vi "Example_OE2031&OE2041 Control.vi"() -> ()   [LabVIEW 2011]
uses:
  <vilib>/Utility/error.llb/DialogType.ctl
panel:
  in  "Sample count":u32
  out "Zero Data?":bool
  in  "buffer":u8
  out "Queue out":errorcluster caption="error out"
  out "Queue output":refnum<queue>
  in  "IP Address":string
  in  "Timeout":u32=100
  in  "Port":u32=10001
  out "Gain Overlaod":bool
  in  "Remote Mode":u16(ring) items=["USB"=0, "RS232"=1, "Ethernet"=3]
  out "Freq":dbl
  out "xita":dbl
  out "R":dbl
  out "Input Overlaod":bool
  out "PLL Lock":bool
  out "Error":string
  out "Serial Versions":string
  in  "Table":T1(tab) caption="选项卡控件"
  in  "OE2041_Configure Input Filter":T2 {"Input Impedance" items=["50Ω", "10MΩ"]; "Input Coupling" items=["AC", "DC"]; "Input Shield Grounding" items=["Float", "Ground"]; "Input Source" items=["A", "B"]}
  in  "OE2041_Configure Ref Phase":T3={"Reference Source"=0, "Sweep Mode"=0, "Start Frequency"=1000.0, "Stop Frequency"=5000.0, "Linear Step Frequency"=1000.0, "Log Step Percent"=10.0, "Step Time(ms)"=1000, "Sweep Run Mode"=0, "Internal Frequency"=1000.0, "Phase  (degree)"=0.0, "External Ref Trigger"=0, "Instrument Mode "=8} {"Instrument Mode" items=["OE2031-10M"=6, "OE2041-30M"=7, "OE2041-60M"=8]; "External Ref Trigger" items=["TTL Rising Edge", "Sine Zero Crossing"]; "Phase  (degree)" min=-180.0 max=180.0 format="%#.2g"; "Internal Frequency" min=1e-05 max=60000000.0 format="%#.3f"; "Sweep Run Mode" items=["Stop", "Singal", "Loop"]; "Log Step Percent" min=-100.0 max=100.0 format="%#.2f"; "Linear Step Frequency" min=1e-05 max=60000000.0 format="%#.3f"; "Stop Frequency" min=1e-05 max=60000000.0 format="%#.3f"; "Start Frequency" min=1e-05 max=60000000.0 format="%#.3f"; "Sweep Mode" items=["Linear", "Log"]; "Reference Source" items=["External", "Internal", "Internal Sweep", "Self"]}
  in  "OE2041_Configure Sens and Filter":T4={"Input Range"=0, "Sensitivity "=24, "Time Constant "=20, "Low Pass Filter Slope "=3, "Enable Sync Filter "=0} {"Enable Sync Filter" items=["OFF", "ON"]; "Low Pass Filter Slope" items=["6 dB/oct", "12 dB/oct", "18 db/oct", "24 dB/oct", "30 dB/oct", "36 dB/oct", "42 dB/oct", "48 dB/oct"]; "Time Constant" items=["30 ns", "60 ns", "125 ns", "250 ns", "500 ns", "1 us", "2 us", "4 us", "8 us", "16 us", "32 us", "64 us", "125 us", "250 us", "500 us", "1 ms", "2 ms", "4 ms", "8 ms", "16 ms", "32 ms", "65 ms", "125 ms", "250 ms", "500 ms", "1 s", "2 s", "4 s", "8 s", "17 s", "35 s", "70 s", "140 s", "275 s", "550 s", "1100 s", "2200 s", "4400 s"]; "Sensitivity" items=["1 nV/fA", "2 nV/fA", "5 nV/fA", "10 nV/fA", "20 nV/fA", "50 nV/fA", "100 nV/fA", "200 nV/fA", "500 nV/fA", "1 uV/pA", "2 uV/pA", "5 uV/pA", "10 uV/pA", "20 uV/pA", "50 uV/pA", "100 uV/pA", "200 uV/pA", "500 uV/pA", "1 mV/nA", "2 mV/nA", "5 mV/nA", "10 mV/nA", "20 mV/nA", "50 mV/nA", "100 mV/nA", "200 mV/nA", "500 mV/nA", "1 V/uA"]; "Input Range" items=["1V", "200mV", "50mV", "10mV", "2mV", "400uV"]}
  in  "OE2041_Configure Channel Out":T5={"parameter"=0, "Speed"=0, "Offset(%)"=0.0, "Expand"=1.0, "AUX OUT"=1.0, "Channel"=0} {"Channel" items=["CH1", "CH2", "CH3", "CH4"]; "AUX OUT" min=-10.0 max=10.0 format="%#.3g"; "Expand" min=1.0 max=256.0 format="%#_3g"; "Offset(%)" min=-100.0 max=100.0 format="%#_5g"; "Speed" items=["Slow", "Fast"]; "parameter" items=["AUXOUT", "X", "Y", "R", "Theta", "Xh1", "Yh1", "Rh1", "Theta h1", "Xh2", "Yh2", "Rh2", "Theta h2", "Xh3", "Yh3", "Rh3", "Theta h3", "X_Noise", "Y_Noise", "Frequency", "AUX-IN1", "AUX-IN2", "AUX-IN3", "AUX-IN4"]}
  in  "OE2041_Configure Sine Out":T6={"Start Value(V)"=0.1, "Sine Output Amplitude (V)"=1.0, "Stop Valve(V)"=1.0, "Sine Step Valve(V)"=0.1, "Step Time(ms) "=1000, "Sine Step Percent(%)"=10.0, "SineOut Mode"=0, "Sine Run Mode"=0, "ADD Mode"=0} {"ADD Mode" items=["OFF", "ON"]; "Sine Run Mode" items=["Stop", "Single", "Loop"]; "SineOut Mode" items=["OFF", "Fixed", "Linear", "Log"]; "Sine Step Percent(%)" min=0.0 max=100.0 format="%#.2g"; "Step Time(ms)" min=1 max=100000; "Sine Step Valve(V)" min=1e-06 max=1.0 format="%#.3g"; "Stop Valve(V)" min=1e-06 max=1.0 format="%#.3g"; "Sine Output Amplitude (V)" min=0.001 max=1.0 format="%#.3g"; "Start Value(V)" min=1e-06 max=1.0 format="%#.3g"}
  in  "OE2041_Configure Demodulator":T7={"A"=1, "F1"=1.0, "B"=1, "F2"=1.0, "Demodulator"=1, "Mode"=0, "Arbitrary Frequency"=1000.0, "Harmonic"=1, "Instrument Mode "=8} {"Instrument Mode" items=["OE2031-10M"=6, "OE2041-30M"=7, "OE2041-60M"=8]; "Harmonic" min=1 max=32767; "Arbitrary Frequency" min=1e-05 max=60000000.0 format="%#.3f"; "Mode" items=["Harm", "Arb_Freq", "Equation"]; "Demodulator" items=["1", "2", "3"]; "F2" min=1e-05 max=60000000.0 format="%#.3g"; "B" min=-32767; "F1" min=1e-05 max=60000000.0 format="%#.3g"; "A" min=-32767}
  in  "OE2041_Auto Setting":T8
  in  "Save Button":bool
  in  "file path":path
  in  "Sample Rate":dbl=0.1 min=0.001 max=100.0
  out "Status":string
  in  "Connect":bool
  in  "VISA resource name":refnum<visa-resource-name>
  in  "Baud Rate (921600)":u32=921600
  # "Tel          :   +86-020-84133345\nWebsite  :   www.ssi-instrument.com\nE-mail     :   support@si-instrument.com"
  # "E="
  # "×"
  # "+"
  # "×"
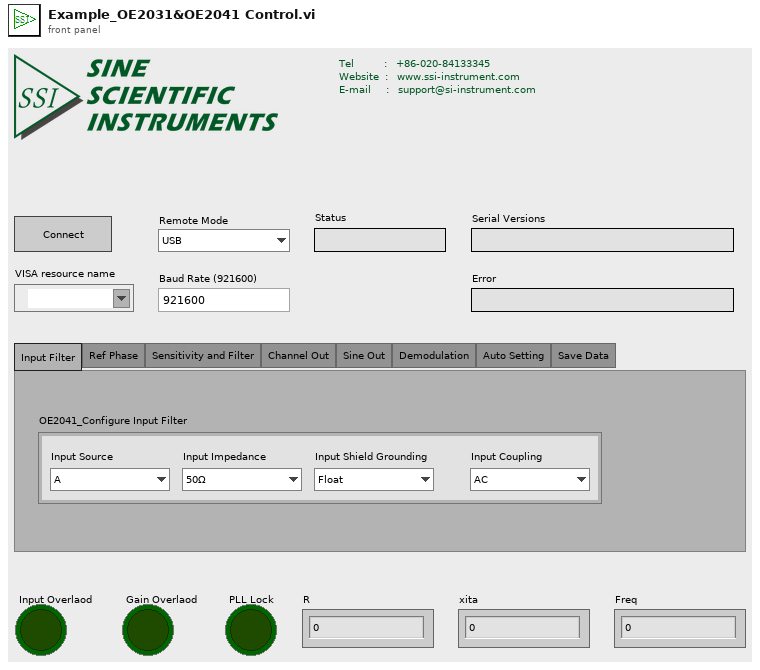
[diagram p1: front panel]
types:
  T1 = enum32{"Input Filter", "Ref Phase", "Sensitivity and Filter", "Channel Out", "Sine Out", "Demodulation", "Auto Setting", "Save Data"}
  T2 = cluster{"Input Source":u16, "Input Shield Grounding ":u16, "Input Coupling ":u16, "Input Impedance ":u16}
  T3 = cluster{"Reference Source":u16, "Sweep Mode":u16, "Start Frequency":dbl, "Stop Frequency":dbl, "Linear Step Frequency":dbl, "Log Step Percent":dbl, "Step Time(ms)":i32, "Sweep Run Mode":u16, "Internal Frequency":dbl, "Phase  (degree)":dbl, "External Ref Trigger":u16, "Instrument Mode ":u16}
  T4 = cluster{"Input Range":u16, "Sensitivity ":u16, "Time Constant ":u8, "Low Pass Filter Slope ":u8, "Enable Sync Filter ":u16}
  T5 = cluster{"parameter":u16, "Speed":u16, "Offset(%)":dbl, "Expand":dbl, "AUX OUT":dbl, "Channel":u16}
  T6 = cluster{"Start Value(V)":dbl, "Sine Output Amplitude (V)":dbl, "Stop Valve(V)":dbl, "Sine Step Valve(V)":dbl, "Step Time(ms) ":u32, "Sine Step Percent(%)":dbl, "SineOut Mode":u8, "Sine Run Mode":u8, "ADD Mode":u8}
  T7 = cluster{"A":i16, "F1":dbl, "B":i16, "F2":dbl, "Demodulator":u16, "Mode":u16, "Arbitrary Frequency":dbl, "Harmonic":u16, "Instrument Mode ":u16}
  T8 = cluster{"Auto Gain":bool, "Auto Phase":bool, "Auto Scale":bool}
  T9 = enum16{"OE1022", "OE1022D", "OE1201", "OE2031&OE2041", "OE1311&OE1351"}
  T10 = cluster{"Port":u32, "Timeout":u32, "IP Address":string}
  T11 = cluster{"PLL Lock(1: External Lock)":bool, "Input Overlaod":bool, "Gain Overlaod":bool}
  T12 = cluster{"X":dbl, "Y":dbl, "R":dbl, "θ":dbl, "Frequency":dbl, "XD1":dbl, "YD1":dbl, "RD1":dbl, "θD1":dbl, "XD2":dbl, "YD2":dbl, "RD2":dbl, "θD2":dbl, "XD3":dbl, "YD3":dbl, "RD3":dbl, "θD3":dbl, "X-Noise":dbl, "Y-Noise":dbl, "AUX-IN1":dbl, "AUX-IN2":dbl, "AUX-IN3":dbl, "AUX-IN4":dbl}
  T13 = typedef "DialogType.ctl" = u16
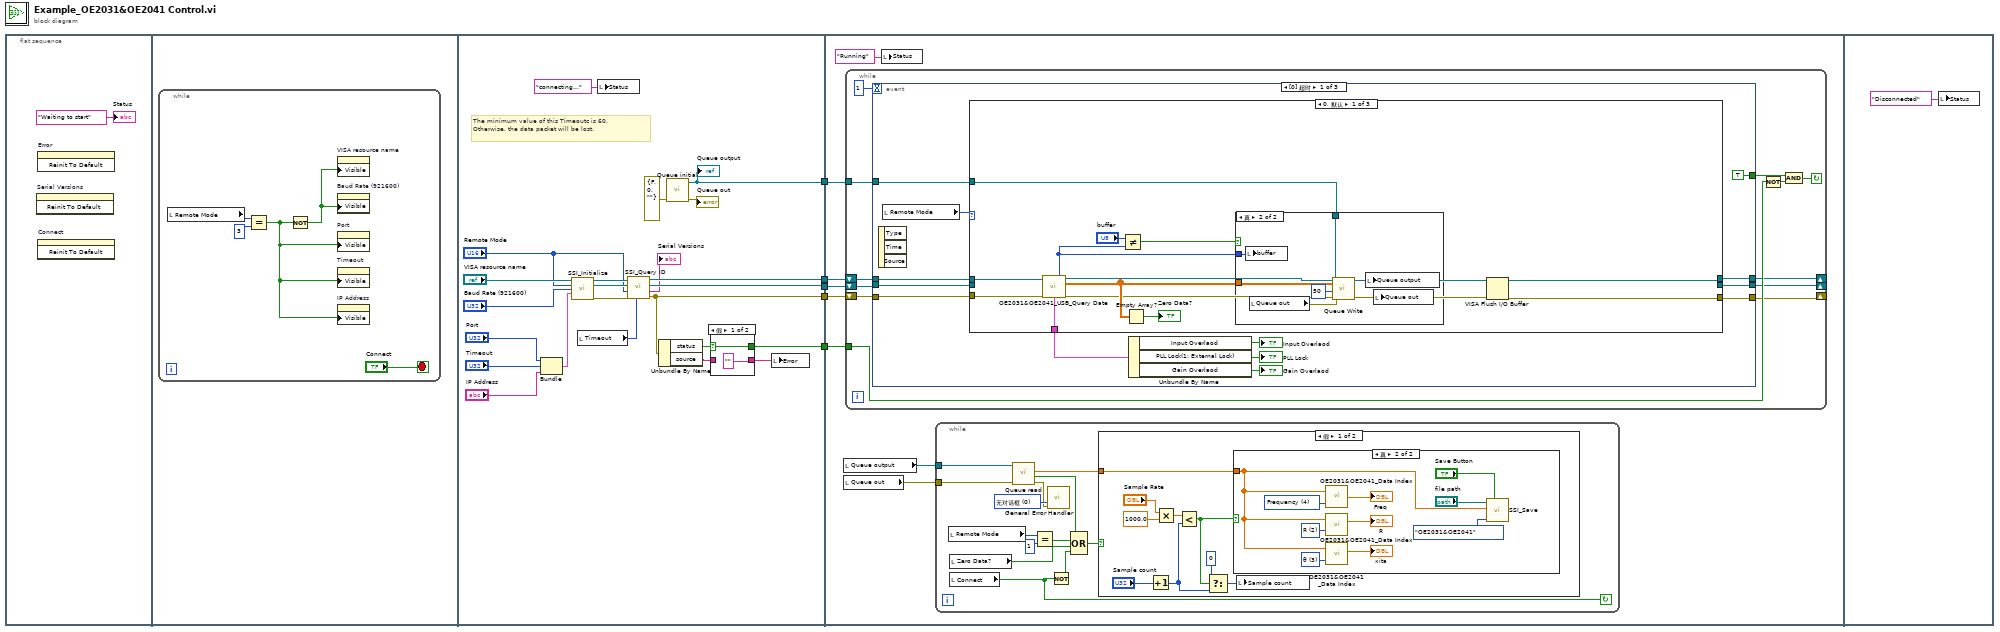
[diagram p0: block diagram]
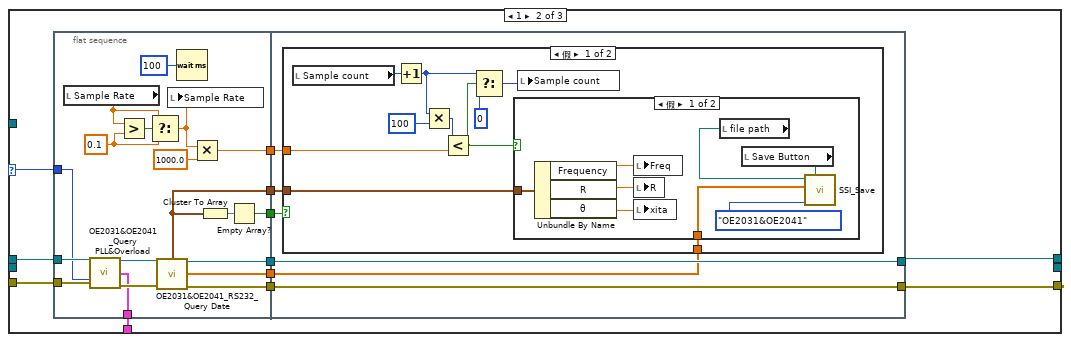
[diagram p6: hidden frame]
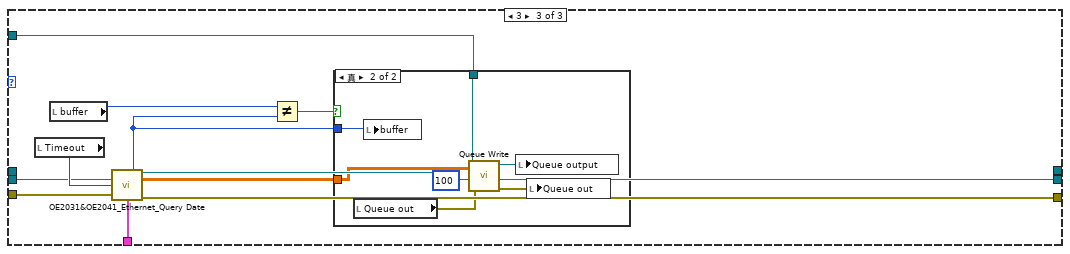
[diagram p9: hidden frame]
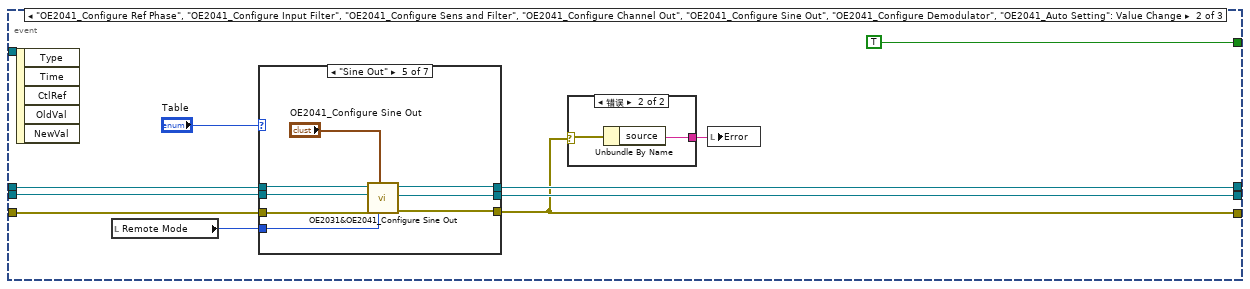
[diagram p11: hidden frame]
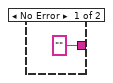
[diagram p12: hidden frame]
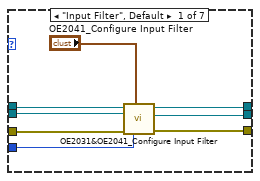
[diagram p13: hidden frame]
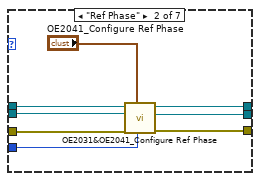
[diagram p14: hidden frame]
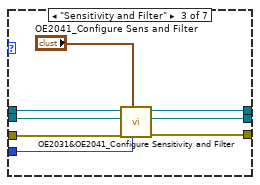
[diagram p15: hidden frame]
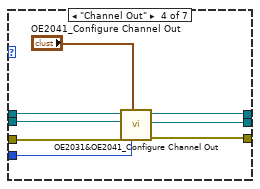
[diagram p16: hidden frame]
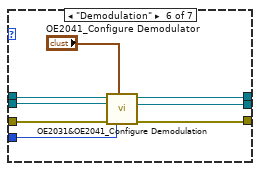
[diagram p17: hidden frame]
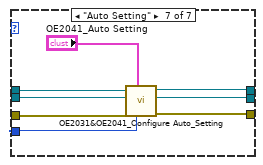
[diagram p18: hidden frame]
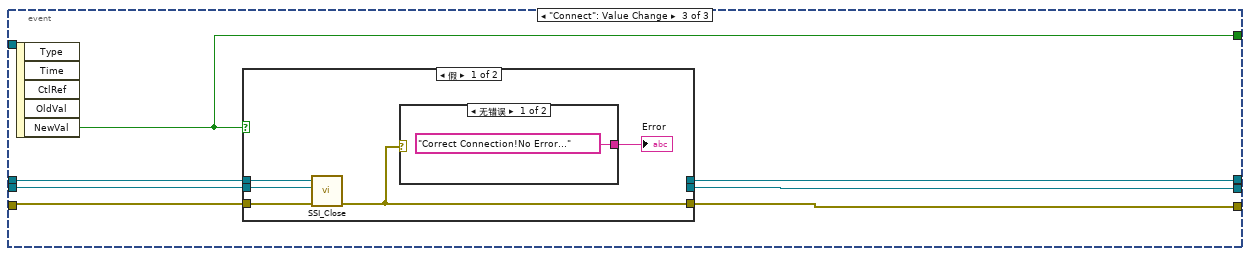
[diagram p19: hidden frame]
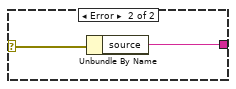
[diagram p20: hidden frame]
diagram:
  n1 = flat-sequence {
    tunnel: [w28] -> w5
    tunnel: [w27] -> w4
    tunnel: [w24] -> w3
    tunnel: [w21] -> w2
    tunnel: [w12] -> w1
    tunnel: w5 -> [w45]
    tunnel: w4 -> [w44]
    tunnel: w3 -> [w43]
    tunnel: w2 -> [w42]
    tunnel: w1 -> [w39]
    frame #0 {
      n2 = invoke on="Serial Versions" class="Str" method="Reinit To Default"() -> ()  [unwired: 3 in, 3 out]
      n3 = invoke on="Error" class="Str" method="Reinit To Default"() -> ()  [unwired: 3 in, 3 out]
      n4 = invoke on="Connect" class="Bool (严格)" method="Reinit To Default"() -> ()  [unwired: 3 in, 3 out]
      "Status" <- "Waiting to start" ("status")
    }
    frame #1 {
      n5 = while {
        stop <- "Connect" stop-if-true
        n6 = local read "Remote Mode"() -> (w10:u16)
        n7 = Equal?(x=w10, y=u16 3) -> (x = y?=w7:bool)
        n8 = Not(x=w7) -> (.not. x?=w8:bool)
        n9 = property on="VISA resource name" class="VISAName"("Visible"=w8) -> ()  [unwired: 2 in, 2 out]
        n10 = property on="Baud Rate (921600)" class="DigNum (严格)"("Visible"=w8) -> ()  [unwired: 2 in, 2 out]
        n11 = property on="Port" class="DigNum (严格)"("Visible"=w7) -> ()  [unwired: 2 in, 2 out]
        n12 = property on="Timeout" class="DigNum (严格)"("Visible"=w7) -> ()  [unwired: 2 in, 2 out]
        n13 = property on="IP Address" class="Str"("Visible"=w7) -> ()  [unwired: 2 in, 2 out]
      }
    }
    frame #2 {
      # "The minimum value of this Timeoutc is 60. \nOtherwise, the data packet will be lost."
      n14 = Bundle("Port"="Port", "Timeout"="Timeout", "IP Address"="IP Address") -> (w16:T10)  [unwired: 1 in]
      n15 = call "SSI_Initialize.vi"("VISA resource name"="VISA resource name", "Remote Mode"="Remote Mode", "baud rate (921600)"="Baud Rate (921600)", "Ethernet"=w16) -> ("VISA resource name out"=w32:refnum<visa-resource-name>, "connection ID(Ethernet)"=w31:refnum<k5>, "error out"=w30:errorcluster)  [unwired: 9 in]
      n16 = local read "Timeout"() -> (w15:u32)
      n17 = local write "Status"("connecting..." ("status")) -> ()
      n18 = call "SSI_Query ID.vi"("Timeout"=w15, "Error in (no error)"=w30, "Remote Mode"="Remote Mode", "Connection ID in"=w31, "VISA resource name"=w32) -> ("Error out"=w24:errorcluster, "Read Buffer"=→"Serial Versions":string, "Connection ID out"=w27:refnum<k5>, "VISA resource  out"=w28:refnum<visa-resource-name>)  [unwired: 3 in]
      n19 = Unbundle By Name(w24) -> ("status"=w23:bool, "source"=w22:string)
      n20 = call "Queue initial.vi"("Error in (no error)"=errorcluster {"status"=FALSE, "code"=0, "source"=""}) -> ("Error out"=→"Queue out":errorcluster, "Queue output"=w12:refnum<queue>)  [unwired: 9 in]
      "Queue output" <- w12
      n21 = case shown="假" w23 {
        selector: w23 -> [w36 w38]
        tunnel: [w36 w38] -> w21
        tunnel: ["" w37] -> w20
        tunnel: w22 -> [_ w37]
        frame False {
        }
        frame True {
        }
      }
      n22 = local write "Error"(w20) -> ()
    }
    frame #3 {
      n23 = local read "Queue output"() -> (w41:refnum<queue>)
      n24 = local read "Queue out"() -> (w40:errorcluster)
      n25 = while {
        tunnel: w42 -> [w86]
        tunnel: w39 -> [w82]
        shift-right: [w79] -> _
        shift-left: w43 -> [w83]
        shift-right: [w80] -> _
        shift-left: w44 -> [w84]
        shift-right: [w81] -> _
        shift-left: w45 -> [w85]
        stop <- w87 continue-if-true
        n26 = event shown="[0] 超时" {
          selector: _ -> [_ _ _]
          dyn-events: _ -> [_ _ _]
          timeout: 1 -> [_ _ _]
          tunnel: [TRUE ("Stop") TRUE ("Stop") w266] -> w88
          tunnel: [w103 w197 w269] -> w79
          tunnel: [w102 w202 w268] -> w81
          tunnel: [w101 w201 w267] -> w80
          tunnel: w85 -> [w94 w205 w272]
          tunnel: w84 -> [w91 w204 w271]
          tunnel: w83 -> [w93 w203 w270]
          tunnel: w82 -> [w95 _ _]
          event Timeout {
            n27 = event-data() -> ()  [unwired: 1 in, 3 out]
            n28 = local read "Remote Mode"() -> (w99:u16)
            n29 = case shown="0, 默认" w99 {
              selector: w99 -> [_ w131 _]
              tunnel: [w107 w133 w187] -> w103
              tunnel: [w108 w132 _] -> w102
              tunnel: [_ _ w188] -> w101
              tunnel: w95 -> [w116 _ w186]
              tunnel: w94 -> [w106 w135 _]
              tunnel: w93 -> [w105 w134 w180]
              tunnel: [w104 w130 w179] -> w92
              tunnel: w91 -> [_ _ w181]
              frame 0, Default {
                n30 = call "OE2031&OE2041_USB_Query Date.vi"("VISA resource name"=w106, "Error in (no error)"=w105) -> ("Buffer Count"=w113:u8, "VISA resource  out"=w110:refnum<visa-resource-name>, "Total Data Array"=w112:dbl[][], "PLL&Overload"=w104:T11, "Error out"=w109:errorcluster)  [unwired: 6 in, 3 out]
                n31 = Not Equal?(x="buffer", y=w113) -> (x != y?=w114:bool)
                n32 = Empty Array?(array=w112) -> (empty?=→"Zero Data?":bool)
                n33 = case shown="真" w114 {
                  tunnel: w112 -> [_ w117]
                  tunnel: w116 -> [_ w122]
                  tunnel: w113 -> [_ w118]
                  frame False {
                  }
                  frame True {
                    n34 = local write "buffer"(w118) -> ()
                    n35 = local read "Queue out"() -> (w119:errorcluster)
                    n36 = call "Queue Write.vi"("Error in (no error)"=w119, "Group Count"=50, "Input Array"=w117, "Queue Input"=w122) -> ("Error out"=w120:errorcluster, "Queue output"=w121:refnum<queue>)  [unwired: 6 in]
                    n37 = local write "Queue output"(w121) -> ()
                    n38 = local write "Queue out"(w120) -> ()
                  }
                }
                n39 = VISA Flush I/O Buffer(VISA resource name=w110, error in (no error)=w109) -> (VISA resource name out=w108:refnum<visa-resource-name>, error out=w107:errorcluster)  [unwired: 1 in]
              }
              frame 1 {
                n40 = flat-sequence {
                  tunnel: [w144] -> w129
                  tunnel: [w145] -> w128
                  tunnel: [w149] -> w127
                  tunnel: [w148] -> w126
                  tunnel: [w143] -> w125
                  tunnel: [w142] -> w124
                  tunnel: [w137] -> w130
                  tunnel: w135 -> [w139]
                  tunnel: w134 -> [w140]
                  tunnel: w131 -> [w138]
                  tunnel: w129 -> [w159]
                  tunnel: w128 -> [w160]
                  tunnel: [w160] -> w132
                  tunnel: [w159] -> w133
                  tunnel: w127 -> [w156]
                  tunnel: w126 -> [w155]
                  tunnel: w125 -> [w157]
                  tunnel: w124 -> [w158]
                  frame #0 {
                    w152 = 0.1 ("y")
                    n41 = local read "Sample Rate"() -> (w147:dbl)
                    n42 = call "OE2031&OE2041_Query PLL&Overload.vi"("VISA resource name"=w139, "Remote Mode"=w138, "Error in (no error)"=w140) -> ("VISA resource  out"=w146:refnum<visa-resource-name>, "OE2041_Query PLL&Overload"=w137:T11, "Error out"=w141:errorcluster)  [unwired: 8 in, 2 out]
                    n43 = Greater?(x=w147, y=w152) -> (0:w151:bool)
                    n44 = Select(t=w147, s=w151, f=w152) -> (s? t:f=w150:dbl)
                    n45 = call "OE2031&OE2041_RS232_Query Date.vi"("VISA resource name"=w146, "Error in (no error)"=w141) -> ("VISA resource  out"=w145:refnum<visa-resource-name>, "Data Array"=w142:dbl[], "Parameter Values"=w143:T12, "Error out"=w144:errorcluster)  [unwired: 9 in, 1 out]
                    n46 = local write "Sample Rate"(w150) -> ()
                    n47 = Wait (ms)(milliseconds to wait=u32 100 ("等待时间（毫秒）")) -> ()  [unwired: 1 out]
                    n48 = Multiply(x=w150, y=1000.0) -> (x*y=w148:dbl)
                    n49 = Cluster To Array(cluster=w143) -> (array=w154:dbl[])
                    n50 = Empty Array?(array=w154) -> (empty?=w149:bool)
                  }
                  frame #1 {
                    n51 = case shown="假" w156 {
                      tunnel: w158 -> [w170 _]
                      tunnel: w157 -> [w169 _]
                      tunnel: w155 -> [w165 _]
                      frame False {
                        n52 = local read "Sample count"() -> (w168:u32)
                        n53 = Increment(x=w168) -> (x+1=w164:u32)
                        n54 = Multiply(x=w164, y=u32 100) -> (x*y=w166:u32)
                        n55 = Less?(x=w166, y=w165) -> (x < y?=w163:bool)
                        n56 = Select(t=w164, s=w163, f=0) -> (s? t:f=w162:u32)
                        n57 = case shown="假" w163 {
                          tunnel: w169 -> [w178 _]
                          tunnel: w170 -> [w174 _]
                          frame False {
                            n58 = Unbundle By Name(w178) -> ("Frequency"=w177:dbl, "R"=w176:dbl, "θ"=w175:dbl)
                            n59 = local write "Freq"(w177) -> ()
                            n60 = local write "R"(w176) -> ()
                            n61 = local write "xita"(w175) -> ()
                            n62 = local read "file path"() -> (w173:path)
                            n63 = local read "Save Button"() -> (w172:bool)
                            n64 = call "SSI_Save.vi"("file path (dialog if empty)"=w173, "1D data"=w174, "Instrument Mode"=T9."OE2031&OE2041", "Save Button"=w172) -> ()  [unwired: 7 in]
                          }
                          frame True {
                          }
                        }
                        n65 = local write "Sample count"(w162) -> ()
                      }
                      frame True {
                      }
                    }
                  }
                }
              }
              frame 3 {
                n66 = local read "Timeout"() -> (w189:u32)
                n67 = local read "buffer"() -> (w184:u8)
                n68 = call "OE2031&OE2041_Ethernet_Query Date.vi"("Connection ID in"=w181, "Timeout"=w189, "Error in (no error)"=w180) -> ("Buffer Count"=w183:u8, "Connection ID out"=w188:refnum<k5>, "Total Data Array"=w182:dbl[][], "PLL&Overload"=w179:T11, "Error out"=w187:errorcluster)  [unwired: 5 in, 3 out]
                n69 = Not Equal?(x=w184, y=w183) -> (x != y?=w185:bool)
                n70 = case shown="真" w185 {
                  tunnel: w186 -> [_ w195]
                  tunnel: w183 -> [_ w191]
                  tunnel: w182 -> [_ w190]
                  frame False {
                  }
                  frame True {
                    n71 = local read "Queue out"() -> (w192:errorcluster)
                    n72 = local write "buffer"(w191) -> ()
                    n73 = call "Queue Write.vi"("Error in (no error)"=w192, "Group Count"=100, "Input Array"=w190, "Queue Input"=w195) -> ("Error out"=w193:errorcluster, "Queue output"=w194:refnum<queue>)  [unwired: 6 in]
                    n74 = local write "Queue output"(w194) -> ()
                    n75 = local write "Queue out"(w193) -> ()
                  }
                }
              }
            }
            n76 = Unbundle By Name(w92) -> ("Input Overlaod"=→"Input Overlaod":bool, "PLL Lock(1: External Lock)"=→"PLL Lock":bool, "Gain Overlaod"=→"Gain Overlaod":bool)
          }
          event "OE2041_Configure Ref Phase", "OE2041_Configure Input Filter", "OE2041_Configure Sens and Filter", "OE2041_Configure Channel Out", "OE2041_Configure Sine Out", "OE2041_Configure Demodulator", "OE2041_Auto Setting": Value Change {
            n77 = event-data() -> ()  [unwired: 1 in, 5 out]
            n78 = local read "Remote Mode"() -> (w200:u16)
            n79 = case shown="\"Sine Out\"" "Table" {
              tunnel: w205 -> [w216 w225 w233 w238 w245 w254 w265]
              tunnel: w204 -> [w215 w224 w231 w239 w244 w255 w264]
              tunnel: w203 -> [w217 w223 w232 w241 w249 w257 w263]
              tunnel: [w212 w222 w229 w235 w246 w253 w261] -> w202
              tunnel: [w213 w221 w230 w237 w248 w252 w259] -> w197
              tunnel: [w214 w220 w228 w236 w247 w251 w260] -> w201
              tunnel: w200 -> [w211 w219 w227 w240 w243 w256 w262]
              frame "Input Filter", Default {
                n80 = call "OE2031&OE2041_Configure Input Filter.vi"("OE2041_Configure Input Filter"="OE2041_Configure Input Filter", "Error in (no error)"=w217, "Remote Mode"=w211, "Connection ID in"=w215, "VISA resource name"=w216) -> ("Error out"=w213:errorcluster, "Connection ID out"=w214:refnum<k5>, "VISA resource  out"=w212:refnum<visa-resource-name>)  [unwired: 3 in, 1 out]
              }
              frame "Ref Phase" {
                n81 = call "OE2031&OE2041_Configure Ref Phase.vi"("OE2041_Configure Ref Phase"="OE2041_Configure Ref Phase", "Error in (no error)"=w223, "Remote Mode"=w219, "Connection ID in"=w224, "VISA resource name"=w225) -> ("Error out"=w221:errorcluster, "Connection ID out"=w220:refnum<k5>, "VISA resource  out"=w222:refnum<visa-resource-name>)  [unwired: 3 in, 1 out]
              }
              frame "Sensitivity and Filter" {
                n82 = call "OE2031&OE2041_Configure Sensitivity and Filter.vi"("OE2041_Configure \nSens and Filter"="OE2041_Configure Sens and Filter", "Error in (no error)"=w232, "Remote Mode"=w227, "Connection ID in"=w231, "VISA resource name"=w233) -> ("Error out"=w230:errorcluster, "Connection ID out"=w228:refnum<k5>, "VISA resource  out"=w229:refnum<visa-resource-name>)  [unwired: 3 in, 1 out]
              }
              frame "Channel Out" {
                n83 = call "OE2031&OE2041_Configure Channel Out.vi"("OE2041_Configure Channel Out"="OE2041_Configure Channel Out", "Error in (no error)"=w241, "Remote Mode"=w240, "Connection ID in"=w239, "VISA resource name"=w238) -> ("Error out"=w237:errorcluster, "Connection ID out"=w236:refnum<k5>, "VISA resource  out"=w235:refnum<visa-resource-name>)  [unwired: 3 in, 1 out]
              }
              frame "Sine Out" {
                n84 = call "OE2031&OE2041_Configure Sine Out.vi"("OE2041_Configure Sine Out"="OE2041_Configure Sine Out", "Error in (no error)"=w249, "Remote Mode"=w243, "Connection ID in"=w244, "VISA resource name"=w245) -> ("Error out"=w248:errorcluster, "Connection ID out"=w247:refnum<k5>, "VISA resource  out"=w246:refnum<visa-resource-name>)  [unwired: 3 in, 1 out]
              }
              frame "Demodulation" {
                n85 = call "OE2031&OE2041_Configure Demodulation.vi"("OE2041_Configure Demodulator"="OE2041_Configure Demodulator", "Error in (no error)"=w257, "Remote Mode"=w256, "Connection ID in"=w255, "VISA resource name"=w254) -> ("Error out"=w252:errorcluster, "Connection ID out"=w251:refnum<k5>, "VISA resource  out"=w253:refnum<visa-resource-name>)  [unwired: 3 in, 1 out]
              }
              frame "Auto Setting" {
                n86 = call "OE2031&OE2041_Configure Auto_Setting.vi"("OE2041_Auto Setting"="OE2041_Auto Setting", "Error in (no error)"=w263, "Remote Mode"=w262, "Connection ID in"=w264, "VISA resource name"=w265) -> ("Error out"=w259:errorcluster, "Connection ID out"=w260:refnum<k5>, "VISA resource  out"=w261:refnum<visa-resource-name>)  [unwired: 3 in, 1 out]
              }
            }
            n87 = case shown="错误" w197 {
              selector: w197 -> [_ w209]
              tunnel: ["" ("source") w208] -> w198
              frame No Error {
              }
              frame Error {
                n88 = Unbundle By Name(w209) -> ("source"=w208:string)
              }
            }
            n89 = local write "Error"(w198) -> ()
          }
          event "Connect": Value Change {
            n90 = event-data() -> ("NewVal"=w266:bool)  [unwired: 1 in, 4 out]
            n91 = case shown="假" w266 {
              tunnel: w272 -> [w277 w282]
              tunnel: w271 -> [w276 w281]
              tunnel: w270 -> [w275 w283]
              tunnel: [w274 w283] -> w269
              tunnel: [_ w282] -> w268
              tunnel: [_ w281] -> w267
              frame False {
                n92 = call "SSI_Close.vi"("Error in (no error)"=w275, "Connection ID in"=w276, "VISA resource name"=w277) -> ("Error out"=w274:errorcluster)  [unwired: 4 in]
                n93 = case shown="无错误" w274 {
                  selector: w274 -> [_ w280]
                  tunnel: ["Correct Connection!No Error..." ("source") w279] -> w273
                  frame No Error {
                  }
                  frame Error {
                    n94 = Unbundle By Name(w280) -> ("source"=w279:string)
                  }
                }
                "Error" <- w273
              }
              frame True {
              }
            }
          }
        }
        n95 = Not(x=w86) -> (.not. x?=w89:bool)
        n96 = And(x=w88, y=w89) -> (x .and. y?=w87:bool)
      }
      n97 = local write "Status"("Running" ("status")) -> ()
      n98 = while {
        tunnel: w41 -> [w52]
        tunnel: w40 -> [w51]
        stop <- w47 continue-if-true
        w54 = T13 0 items=["无对话框", "确定信息", "继续或停止信息", "确定信息＋警告", "继续/停止+警告"] ("type of dialog (OK msg:1)")
        n99 = local read "Remote Mode"() -> (w59:u16)
        n100 = local read "Zero Data?"() -> (w55:bool)
        n101 = local read "Connect"() -> (w47:bool)
        n102 = call "Queue read.vi"("Error in (no error)"=w51, "Queue Input"=w52) -> ("Error out"=w53:errorcluster, "Timeout？"=w49:bool, "Output Array"=w50:sgl[])  [unwired: 7 in]
        n103 = Equal?(x=w59, y=u16 1) -> (x = y?=w56:bool)
        n104 = call <vilib>:"General Error Handler.vi"("type of dialog (OK msg:1)"=w54, "error in (no error)"=w53) -> ()  [unwired: 9 in, 5 out]
        n105 = Not(x=w47) -> (.not. x?=w48:bool)
        n106 = Compound Arithmetic op=OR(w49, w56, w55, w48) -> (w57:bool)
        n107 = case shown="假" w57 {
          tunnel: w50 -> [w68 _]
          frame False {
            n108 = Increment(x="Sample count") -> (x+1=w62:u32)
            n109 = Multiply(x="Sample Rate", y=1000.0) -> (x*y=w66:dbl)
            n110 = Less?(x=w66, y=w62) -> (x < y?=w63:bool)
            n111 = Select(t=0, s=w63, f=w62) -> (s? t:f=w61:u32)
            n112 = case shown="真" w63 {
              tunnel: w68 -> [_ w70]
              frame False {
              }
              frame True {
                w78 = u16 3 items=["X", "Y", "R", "θ", "Frequency", "XD1", "YD1", "RD1", "θD1", "XD2", "YD2", "RD2", "θD2", "XD3", "YD3", "RD3", "θD3", "X_Noise", "Y_Noise", "AUXADC1", "AUXADC2", "AUXADC3", "AUXADC4"] ("Parameter Type")
                w77 = u16 2 items=["X", "Y", "R", "θ", "Frequency", "XD1", "YD1", "RD1", "θD1", "XD2", "YD2", "RD2", "θD2", "XD3", "YD3", "RD3", "θD3", "X_Noise", "Y_Noise", "AUXADC1", "AUXADC2", "AUXADC3", "AUXADC4"] ("Parameter Type")
                w76 = u16 4 items=["X", "Y", "R", "θ", "Frequency", "XD1", "YD1", "RD1", "θD1", "XD2", "YD2", "RD2", "θD2", "XD3", "YD3", "RD3", "θD3", "X_Noise", "Y_Noise", "AUXADC1", "AUXADC2", "AUXADC3", "AUXADC4"] ("Parameter Type")
                n113 = call "OE2031&OE2041_Data Index.vi"("Parameter Type"=w76, "Input Date Array"=w70) -> ("Parameter"=→"Freq":dbl)
                n114 = call "OE2031&OE2041_Data Index.vi"("Parameter Type"=w77, "Input Date Array"=w70) -> ("Parameter"=→"R":dbl)
                n115 = call "OE2031&OE2041_Data Index.vi"("Parameter Type"=w78, "Input Date Array"=w70) -> ("Parameter"=→"xita":dbl)
                n116 = call "SSI_Save.vi"("file path (dialog if empty)"="file path", "1D data"=w70, "Instrument Mode"=T9."OE2031&OE2041", "Save Button"="Save Button") -> ()  [unwired: 7 in]
              }
            }
            n117 = local write "Sample count"(w61) -> ()
          }
          frame True {
          }
        }
      }
    }
    frame #4 {
      n118 = local write "Status"("Disconnected" ("status")) -> ()
    }
  }
